vi "Update VS channels - outgoing (object info).vi"(8 "object info":T2, 9 "obj key":T1, 10 "out_objectMap in":T3, 11 "values in":dbl[](array[numeric])) -> (2 "out_objectMap out":T3, 3 "values out":dbl[](array[numeric]))   [LabVIEW 2019, in "HLA Custom Device Engine.lvlib"]
uses:
  HLA Custom Device Engine.lvlib
  _typedefs/map_object.ctl
  _typedefs/map_object_key.ctl
  _typedefs/map_object_value.ctl
  _typedefs/map_attr_param_data.ctl
  _typedefs/object_info_outgoing_type.ctl
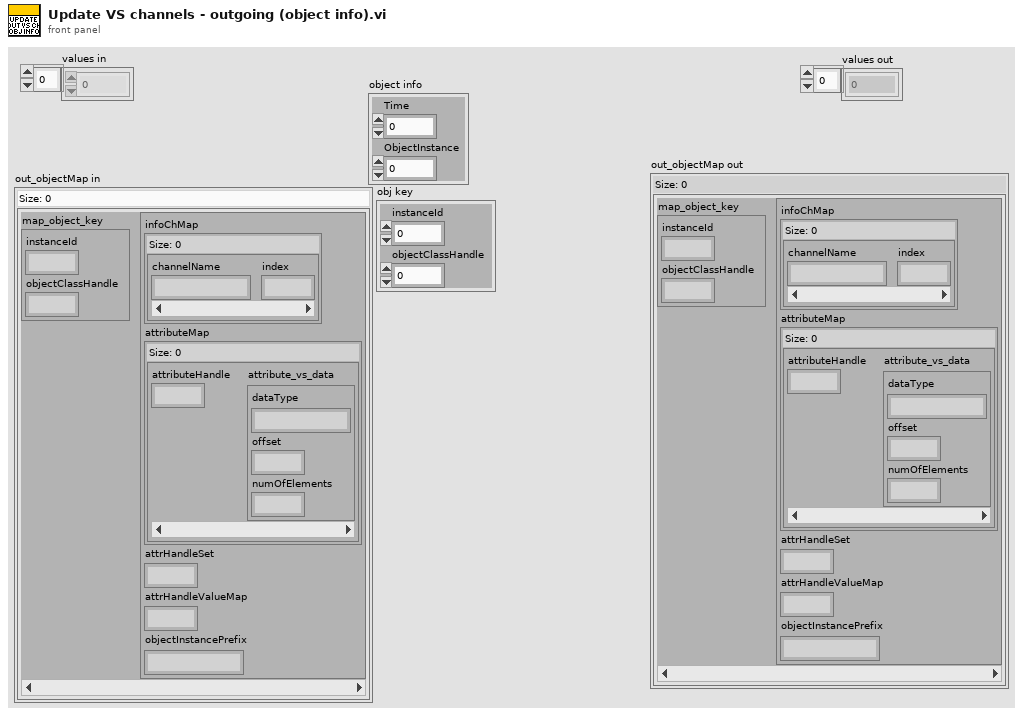
[diagram p1: front panel]
types:
  T1 = typedef "HLA Custom Device Engine.lvlib/map_object_key.ctl" = cluster{"instanceId":i32, "objectClassHandle":u64}
  T2 = typedef "HLA Custom Device Engine.lvlib/object_info_outgoing_type.ctl" = cluster{"Time":dbl, "ObjectInstance":u64}
  T3 = typedef "HLA Custom Device Engine.lvlib/map_object.ctl" = map{T1, T4}
  T4 = typedef "HLA Custom Device Engine.lvlib/map_object_value.ctl" = cluster{"infoChMap":map{string, i32}, "attributeMap":map{u64, T5}, "attrHandleSet":u64, "attrHandleValueMap":u64, "objectInstancePrefix":string}
  T5 = typedef "HLA Custom Device Engine.lvlib/map_attr_param_data.ctl" = cluster{"dataType":string, "offset":i32, "numOfElements":i32}
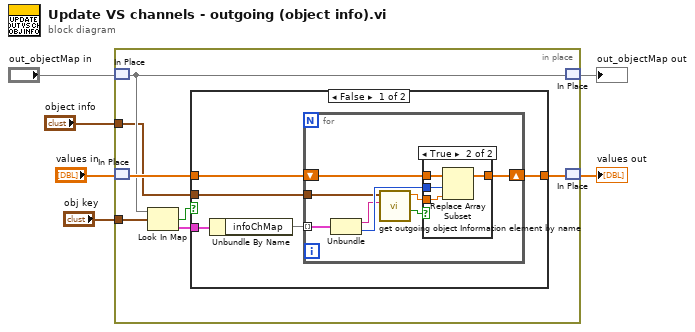
[diagram p0: block diagram]
diagram:
  n1 = in-place {
    in-place-border: "object info" -> [w8]
    in-place-border: "obj key" -> [w7]
    n2 = in-place-match #1("out_objectMap in") -> (w9:T3)
    n3 = in-place-match #2("values in") -> (w11:dbl[])
    n4 = Look In Map(map=w9, key=w7) -> (key not found?=w13:bool, value=w12:T4)  [unwired: 1 in]
    n5 = case shown="False" w13 {
      tunnel: [w17 w32] -> w10
      tunnel: w12 -> [w15 _]
      tunnel: w11 -> [w16 w32]
      tunnel: w8 -> [w14 _]
      frame False {
        n6 = Unbundle By Name(w15) -> ("infoChMap"=w18:map{string, i32})
        n7 = for {
          tunnel: w18 -> [w23] mode=indexing
          shift-right: [w25] -> w17
          shift-left: w16 -> [w26]
          tunnel: w14 -> [w22]
          n8 = Unbundle(w23) -> ("channelName"=w21:string, "index"=w24:i32)
          n9 = call "get outgoing object Information element by name.vi"("name"=w21, "object info"=w22) -> ("found"=w19:bool, "element out"=w20:dbl)  [unwired: 8 in]
          n10 = case shown="True" w19 {
            tunnel: w26 -> [w27 w31]
            tunnel: [w27 w30] -> w25
            tunnel: w24 -> [_ w29]
            tunnel: w20 -> [_ w28]
            frame False {
            }
            frame True {
              n11 = Replace Array Subset(array=w31, new element=w28, index=w29) -> (w30:dbl[])
            }
          }
        }
      }
      frame True {
      }
    }
    n12 = in-place-match #1(w9) -> (→"out_objectMap out":T3)
    n13 = in-place-match #2(w10) -> (→"values out":dbl[])
  }
